vi "AlazarDSPGetParameterU32.vi"(4 "error in (no error)":errorcluster, 5 "Parameter":u32(ring) items=["Raw+FFT supported", "FFT subtractor supported"], 7 "DSP Handle":u64) -> (0 "error out":errorcluster, 1 "Return Code":u32, 2 "result":u32, 3 "DSP Handle":u64)   [LabVIEW 2018]
doc: "Get a device attribute as a signed long value."
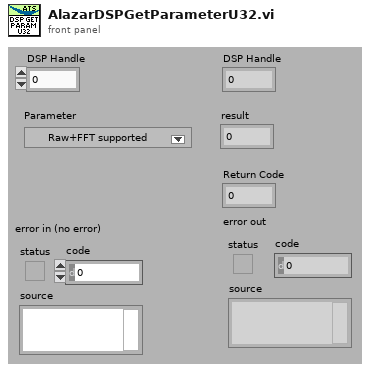
[diagram p1: front panel]
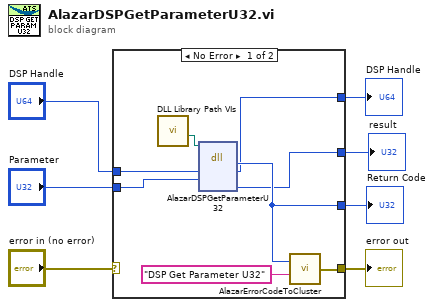
[diagram p0: block diagram]
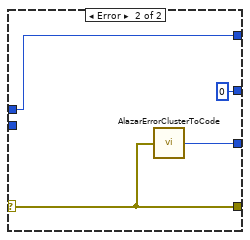
[diagram p2: hidden frame]
diagram:
  n1 = case shown="No Error" "error in (no error)" {
    selector: "error in (no error)" -> [_ w19]
    tunnel: [w12 w19] -> w6
    tunnel: [w14 w18] -> w5
    tunnel: "DSP Handle" -> [w15 w17]
    tunnel: [w11 w17] -> w3
    tunnel: "Parameter" -> [w9 _]
    tunnel: [w10 0] -> w1
    frame No Error {
      n2 = call "DLL Library Path VIs.vi"() -> ("Alazar"=w8:path)  [unwired: 9 in, 2 out]
      n3 = dll-call lib="C:/Project/SerialSectOCT - FFT GPU/SerialSectOCT/Labview Software/DLL/ATSApi.dll" fn="AlazarDSPGetParameterU32"(path in=w8, "dspHandle"=w15, "parameter"=w9) -> ("return type"=w14:u32, "dspHandle"=w11:u64, "result"=w10:u32)  [unwired: 4 in, 2 out]
      n4 = call "AlazarErrorCodeToCluster.vi"("Message"="DSP Get Parameter U32", "Error Code"=w14) -> ("error out"=w12:errorcluster)
    }
    frame Error {
      n5 = call "AlazarErrorClusterToCode.vi"("error in (no error)"=w19) -> ("Error Code"=w18:u32)
    }
  }
  "DSP Handle" <- w3
  "error out" <- w6
  "Return Code" <- w5
  "result" <- w1
